vi "HV Load Test_w_iVIO_Meas.vi"(5 "Published_Data_ID":string="HV_", 7 "Reg0_State":string="State00", 10 "HV_Load_Steps_uA":dbl[](array[numeric])=[0.0, 5.0, 8.0, 10.0] format="%#_6p", 11 "Semiconductor Module Context":T1) -> (0 "error out":errorcluster)   [LabVIEW 2013]
uses:
  <vilib>/NI_TestStand_SemiconductorModule/NI_TestStand_Semiconductor_Module.lvlibp/PinMap/General/SemiconductorModuleContext.ctl
  <vilib>/NI_TestStand_SemiconductorModule/NI_TestStand_Semiconductor_Module.lvlibp/PinMap/DC Power/PinsToNIDCPowerSessions.vi
  <vilib>/NI_TestStand_SemiconductorModule/NI_TestStand_Semiconductor_Module.lvlibp/PinMap/Deprecated/PublishDataDoubleMultiplePinsMultipleInstruments.vi
  <vilib>/NI_TestStand_SemiconductorModule/NI_TestStand_Semiconductor_Module.lvlibp/PinMap/General/Publish/PublishDataDouble2D.vi
  <vilib>/NI_TestStand_SemiconductorModule/NI_TestStand_Semiconductor_Module.lvlibp
panel:
  out "voltage measurements":dbl[][](array[numeric])
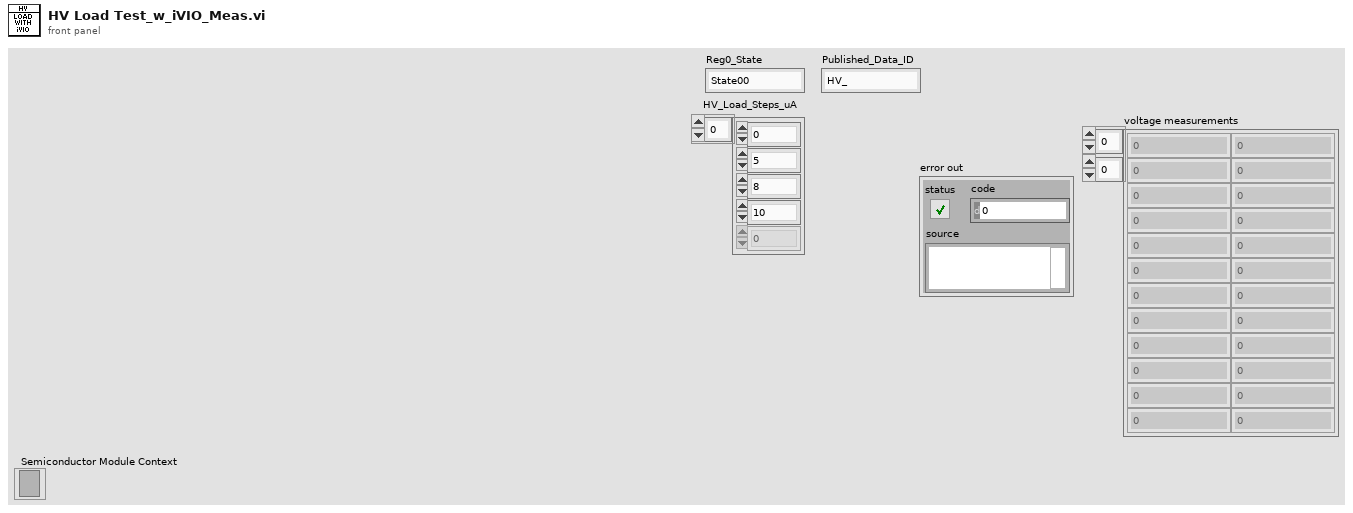
[diagram p1: front panel]
types:
  T1 = typedef "NI_TestStand_Semiconductor_Module.lvlibp/SemiconductorModuleContext.ctl" = refnum<k7>
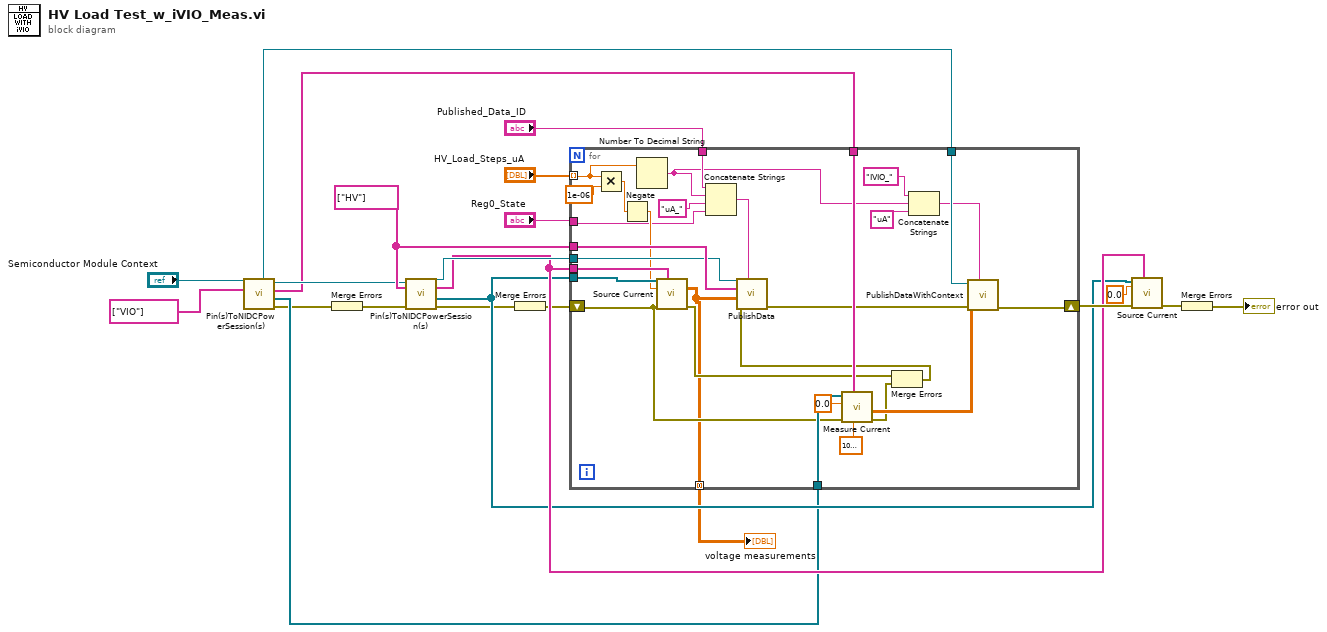
[diagram p0: block diagram]
diagram:
  w18 = string[] ["HV"] ("Pins")
  n1 = call-poly <vilib>:"Pin(s)ToNIDCPowerSession(s).vi"("Pins"=string[] ["VIO"], "Semiconductor Module Context"="Semiconductor Module Context") -> ("error out"=w3:errorcluster, "Instrument Sessions"=w5:refnum<k15>[], "Channel Lists"=w10:string[], "Semiconductor Module Context Out"=w12:T1, "Pin Query Context"=w9:refnum<class "MultiplePinMultipleSessionQueryContext.lvclass">)  [unwired: 5 in]
  n2 = Merge Errors(w3) -> (w8:errorcluster)
  n3 = call-poly <vilib>:"Pin(s)ToNIDCPowerSession(s).vi"("error in (no error)"=w8, "Pins"=w18, "Semiconductor Module Context"=w12) -> ("error out"=w2:errorcluster, "Instrument Sessions"=w7:refnum<k15>[], "Channel Lists"=w15:string[], "Semiconductor Module Context Out"=w22:T1)  [unwired: 4 in, 1 out]
  n4 = Merge Errors(w2) -> (w6:errorcluster)
  n5 = for {
    tunnel: w18 -> [w51]
    tunnel: w22 -> [w50]
    tunnel: w15 -> [w47]
    tunnel: "HV_Load_Steps_uA" -> [w40] mode=indexing
    tunnel: w7 -> [w49]
    shift-right: [w33] -> w19
    shift-left: w6 -> [w28]
    tunnel: "Published_Data_ID" -> [w45]
    tunnel: "Reg0_State" -> [w41]
    tunnel: w10 -> [w38]
    tunnel: w5 -> [w39]
    tunnel: w9 -> [w36]
    tunnel: [w23] -> w1 mode=concatenating
    n6 = Multiply(x=w40, y=1e-06) -> (x*y=w42:dbl)
    n7 = Negate(x=w42) -> (-x=w43:dbl)
    n8 = Number To Decimal String(number=w40) -> (decimal integer string=w37:string)  [unwired: 1 in]
    n9 = call "Source Current.vi"("Channel Lists"=w47, "error in (no error)"=w28, "current level"=w43, "Instrument Sessions In"=w49) -> ("error out"=w26:errorcluster, "voltage measurements"=w23:dbl[][])  [unwired: 4 in, 2 out]
    n10 = Concatenate Strings(w45, w37, "uA_" ("string"), w41) -> (w46:string)
    n11 = call "Measure Current.vi"("Result Multiplier"=1000000.0, "Channel Lists"=w38, "error in (no error)"=w28, "Delay Time (s)"=0.0, "DCPower Sessions In"=w39) -> ("error out"=w27:errorcluster, "current measurements"=w35:dbl[][])  [unwired: 4 in, 1 out]
    n12 = Merge Errors(w26, w27) -> (w25:errorcluster)
    n13 = call-poly <vilib>:"PublishData.vi"("Measurement Id"=w46, "error in (no error)"=w25, "Data In"=w23, "Pins"=w51, "Semiconductor Module Context"=w50) -> ("error out"=w24:errorcluster)  [unwired: 5 in, 1 out]
    n14 = Concatenate Strings("IVIO_" ("string"), w37, "uA" ("string")) -> (w34:string)
    n15 = call-poly <vilib>:"PublishDataWithContext.vi"("Published Data Id"=w34, "error in (no error)"=w24, "Data In"=w35, "Pin Query Context"=w36) -> ("error out"=w33:errorcluster)  [unwired: 6 in, 1 out]
  }
  "voltage measurements" <- w1
  n16 = call "Source Current.vi"("Channel Lists"=w15, "error in (no error)"=w19, "current level"=0.0, "Instrument Sessions In"=w7) -> ("error out"=w4:errorcluster)  [unwired: 4 in, 3 out]
  n17 = Merge Errors(w4) -> (→"error out":errorcluster)
